vi "create_caxis_fine_sweep.vi"(8 "Error In":errorcluster, 9 "Variable to Change":T1, 10 "phic center":dbl, 11 "thetac center":dbl) -> (0 "Error Out":errorcluster, 2 "phic":dbl[](array[numeric]), 3 "thetac":dbl[](array[numeric]))   [LabVIEW 2019]
doc: "Create arrays +/- 5 degrees around the thetac, phic center values (only 1 variable at a time) in 0.01 degree steps. Original program used +/- 2 degrees, but we expanded it for robustness."
uses:
  thetac_phic_enum_typedef.ctl
panel:
  out "phi size":i32
  out "theta size":i32
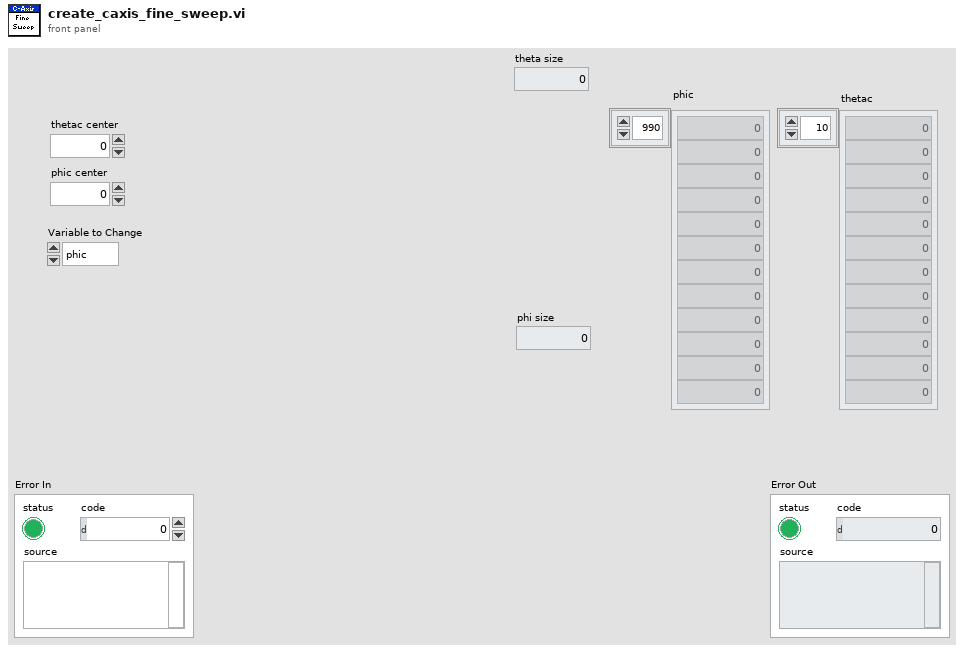
[diagram p1: front panel]
types:
  T1 = typedef "thetac_phic_enum_typedef.ctl" = enum16{"phic", "thetac"}
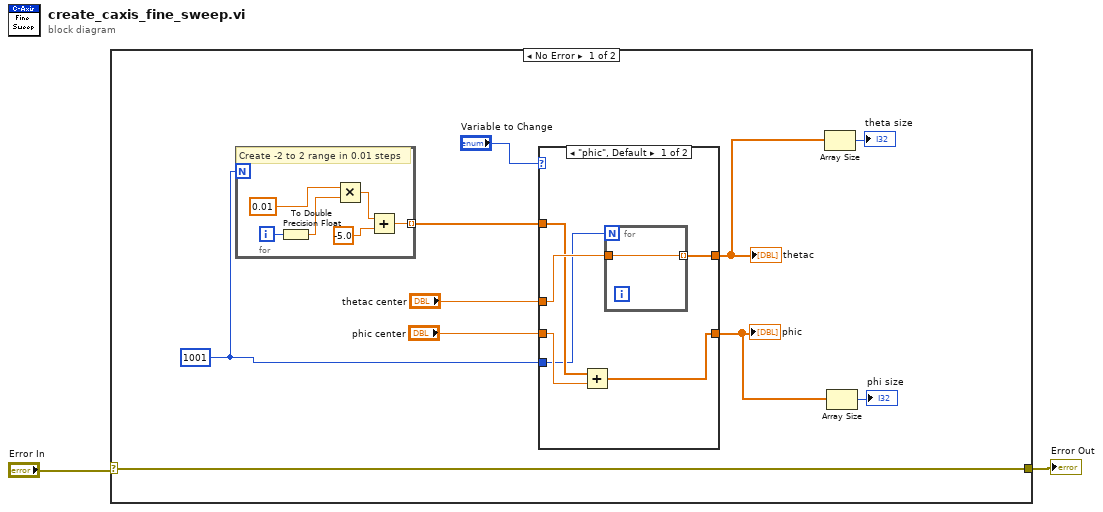
[diagram p0: block diagram]
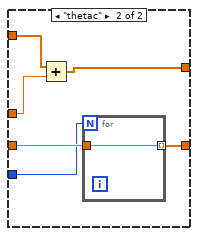
[diagram p2: hidden frame]
diagram:
  n1 = case shown="No Error" "Error In" {
    selector: "Error In" -> [w12 w33]
    tunnel: [w12 w33] -> w1
    frame No Error {
      w3 = 1001
      n2 = for {
        N: w3 -> [_]
        tunnel: [w27] -> w10 mode=indexing
        i -> [w31]
        # "Create -2 to 2 range in 0.01 steps"
        n3 = To Double Precision Float(number=w31) -> (double precision float=w30:dbl)
        n4 = Multiply(x=0.01, y=w30) -> (x*y=w29:dbl)
        n5 = Add(x=w29, y=-5.0 ("x*y")) -> (x+y=w27:dbl)
      }
      n6 = case shown="\"phic\", Default" "Variable to Change" {
        tunnel: w10 -> [w14 w25]
        tunnel: "thetac center" -> [w18 w24]
        tunnel: "phic center" -> [w15 w22]
        tunnel: [w17 w23] -> w7
        tunnel: [w16 w21] -> w4
        tunnel: w3 -> [w13 w20]
        frame "phic", Default {
          n7 = Add(x=w14, y=w15) -> (x+y=w16:dbl[])
          n8 = for {
            N: w13 -> [_]
            tunnel: w18 -> [w19]
            tunnel: [w19] -> w17 mode=indexing
          }
        }
        frame "thetac" {
          n9 = Add(x=w25, y=w24) -> (x+y=w23:dbl[])
          n10 = for {
            N: w20 -> [_]
            tunnel: w22 -> [w26]
            tunnel: [w26] -> w21 mode=indexing
          }
        }
      }
      "phic" <- w4
      "thetac" <- w7
      n11 = Array Size(array=w7) -> (size(s)=→"theta size":i32)
      n12 = Array Size(array=w4) -> (size(s)=→"phi size":i32)
    }
    frame Error {
    }
  }
  "Error Out" <- w1
